vi "Outer Product PtByPt.vi"(0 "y":dbl format="%0.2f", 1 "sample length y":i32=10, 2 "x":dbl format="%0.2f", 3 "sample length x":i32=10, 4 "initialize":bool) -> (5 "Outer Product":dbl[][](array[numeric]), 6 "error":i32)   [LabVIEW 2017, in "NI_PtbyPt.lvlib"]
doc: "Computes the <B>Outer Product</B> of <B>y</B> and <B>x</B>."
uses:
  <vilib>/ptbypt/NI_PtbyPt.lvlib
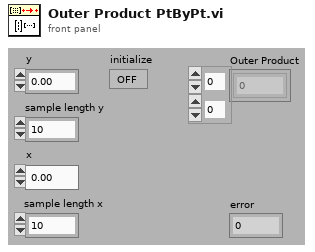
[diagram p1: front panel]
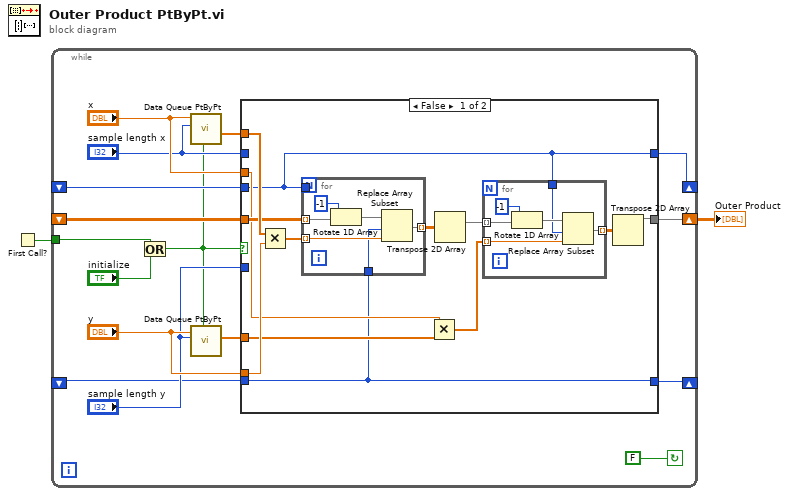
[diagram p0: block diagram]
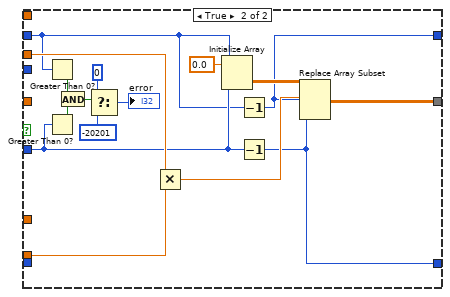
[diagram p2: hidden frame]
diagram:
  n1 = First Call?() -> (First Call?: T/F=w1:bool)
  n2 = while {
    tunnel: w1 -> [w5]
    shift-left: _ -> [w7]
    shift-right: [w8] -> _
    shift-left: _ -> [w10]
    shift-right: [w11] -> _
    shift-left: _ -> [w18]
    shift-right: [w17] -> w2
    stop <- FALSE continue-if-true
    n3 = Or(x=w5, y="initialize") -> (x .or. y?=w3:bool)
    n4 = call <vilib>:"Data Queue PtByPt.vi"("initialize"=w3, "sample length"="sample length x", "input data point"="x") -> ("Previous Queue"=w12:dbl[])  [unwired: 4 in, 4 out]
    n5 = call <vilib>:"Data Queue PtByPt.vi"("initialize"=w3, "sample length"="sample length y", "input data point"="y") -> ("Current Queue"=w9:dbl[])  [unwired: 4 in, 4 out]
    n6 = case shown="False" w3 {
      tunnel: w18 -> [w29 _]
      tunnel: [w21 w54] -> w17
      tunnel: "x" -> [w24 w59]
      tunnel: "y" -> [w31 w58]
      tunnel: "sample length y" -> [_ w53]
      tunnel: "sample length x" -> [_ w46]
      tunnel: w12 -> [w30 _]
      tunnel: [w19 w44] -> w11
      tunnel: w10 -> [w19 _]
      tunnel: w9 -> [w25 _]
      tunnel: [w20 w45] -> w8
      tunnel: w7 -> [w20 _]
      frame False {
        n7 = Multiply(x=w30, y=w31) -> (x*y=w28:dbl[])
        n8 = for {
          tunnel: w29 -> [w43] mode=indexing
          tunnel: w19 -> [_]
          tunnel: w28 -> [w40] mode=indexing
          tunnel: [w39] -> w27 mode=indexing
          tunnel: w20 -> [w38]
          n9 = Rotate 1D Array(1:w43, 2:-1) -> (0:w41:dbl[])
          n10 = Replace Array Subset(array=w41, new element=w40, index=w38) -> (w39:dbl[])
        }
        n11 = Multiply(x=w24, y=w25) -> (x*y=w23:dbl[])
        n12 = Transpose 2D Array(2D array=w27) -> (transposed array=w26:dbl[][])
        n13 = for {
          tunnel: w26 -> [w37] mode=indexing
          tunnel: w23 -> [w34] mode=indexing
          tunnel: [w33] -> w22 mode=indexing
          tunnel: w19 -> [w32]
          n14 = Rotate 1D Array(1:w37, 2:-1) -> (0:w35:dbl[])
          n15 = Replace Array Subset(array=w35, new element=w34, index=w32) -> (w33:dbl[])
        }
        n16 = Transpose 2D Array(2D array=w22) -> (transposed array=w21:dbl[][])
      }
      frame True {
        n17 = Greater Than 0?(x=w46) -> (x > 0?=w52:bool)
        n18 = Greater Than 0?(x=w53) -> (x > 0?=w51:bool)
        n19 = And(x=w52, y=w51) -> (x .and. y?=w50:bool)
        n20 = Select(t=0, s=w50, f=-20201) -> (s? t:f=→"error":i32)
        n21 = Multiply(x=w59, y=w58) -> (x*y=w55:dbl)
        n22 = Initialize Array(0.0 ("Element Data"), w46, w53) -> (w56:dbl[][])
        n23 = Decrement(x=w46) -> (x-1=w44:i32)
        n24 = Decrement(x=w53) -> (x-1=w45:i32)
        n25 = Replace Array Subset(array=w56, new element=w55, index (row)=w44, index (col)=w45) -> (w54:dbl[][])
      }
    }
  }
  "Outer Product" <- w2
